vi "读取外设配置.vi"(8 "error in (no error)":errorcluster, 11 "MB session in":refnum<class "MB_Master.lvclass">) -> (0 "error out":errorcluster, 2 "外设配置":T1 {"光谱仪类型" items=["1型", "2型"]; "泵阀量" items=["9通"=9, "12通"=12]; "泵类型" items=["1型", "2型"]}, 3 "MB session out":refnum<class "MB_Master.lvclass">)   [LabVIEW 2016, in "斯坦道总磷总氮.lvlib"]
uses:
  <vilib>/Plasmionique/MB Master/MB_Master/MB_Master.lvclass
  <vilib>/Plasmionique/MB Master/MB_Master_Serial/MB_Master_Serial.lvclass
  C:/Program Files (x86)/National Instruments/LabVIEW 2016/vi.lib/Plasmionique/MB Master/MB_Master/MB_Master.lvclass
  <vilib>/Plasmionique/MB Master/MB Master.lvlib
panel:
  in  "VISA Resource":refnum<visa-resource-name>
  in  "引用选择":enum16{"MB引用", "自建引用"}(ring)
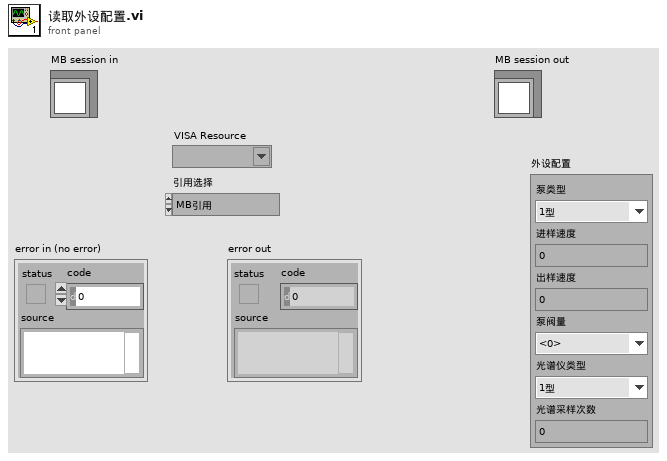
[diagram p1: front panel]
types:
  T1 = cluster{"泵类型":u16, "进样速度":u32, "出样速度":u32, "泵阀量":u16, "光谱仪类型":u16, "光谱采样次数":u8}
  T2 = cluster{"baud rate (bps)":u32, "stop bits":u16, "parity":u16, "flow control":u16, "timeout":u32, "retries":i32}
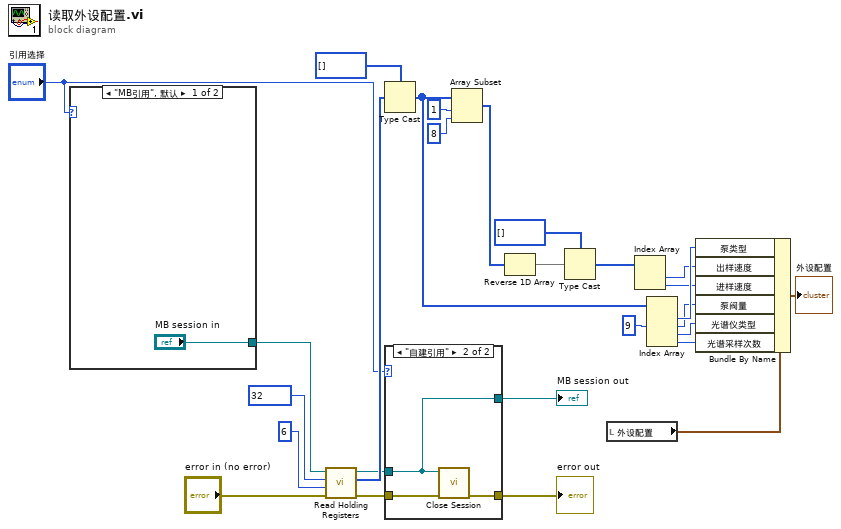
[diagram p0: block diagram]
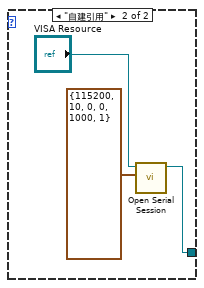
[diagram p3: hidden frame]
diagram:
  n1 = case shown="\"MB引用\", 默认" "引用选择" {
    tunnel: ["MB session in" w31] -> w7
    frame "MB引用", Default {
    }
    frame "自建引用" {
      n2 = call <vilib>:"Open Serial Session.vi"("Serial Config"=T2 {"baud rate (bps)"=115200, "stop bits"=10, "parity"=0, "flow control"=0, "timeout"=1000, "retries"=1}, "VISA Resource"="VISA Resource") -> ("MB_Serial session"=w31:refnum<class "MB_Master_Serial.lvclass">)  [unwired: 8 in, 1 out]
    }
  }
  n3 = call <vilib>:"Read Holding Registers.vi"("error in (no error)"="error in (no error)", "quantity"=u16 6, "starting address"=u16 32, "MB session in"=w7) -> ("error out"=w3:errorcluster, "Registers"=w24:u16[], "MB session out"=w6:refnum<class "MB_Master.lvclass">)  [unwired: 5 in]
  n4 = Type Cast(type=u8[] [], x=w24) -> (*(type *) &x=w19:u8[])
  n5 = case shown="\"自建引用\"" "引用选择" {
    tunnel: w6 -> [w32 w34]
    tunnel: w3 -> [w33 w36]
    tunnel: [w33 w35] -> w2
    tunnel: [w32 w34] -> w1
    frame "MB引用", Default {
    }
    frame "自建引用" {
      n6 = call-dynamic "Close Session.vi"("error in (no error)"=w36, "MB session in"=w34) -> ("error out"=w35:errorcluster)  [unwired: 9 in]
    }
  }
  "MB session out" <- w1
  "error out" <- w2
  n7 = Array Subset(array=w19, index=1 ("索引"), length=8 ("长度")) -> (w16:u8[])
  n8 = Reverse 1D Array(array=w16) -> (reversed array=w15:u8[])
  n9 = Type Cast(type=u32[] [], x=w15) -> (*(type *) &x=w13:u32[])
  n10 = local read "外设配置"() -> (w22:T1)
  n11 = Index Array(array=w13) -> (element #1=w12:u32, element #2=w11:u32)  [unwired: 2 in]
  n12 = Index Array(array=w19, index #2=9 ("索引")) -> (element #1=w20:u8, element #2=w9:u8, element #3=w8:u8, element #4=w5:u8)  [unwired: 3 in]
  n13 = Bundle By Name(cluster=w22, "泵类型"=w20, "出样速度"=w12, "进样速度"=w11, "泵阀量"=w9, "光谱仪类型"=w8, "光谱采样次数"=w5) -> (→"外设配置":T1)
